vi "RGseriesSeria210216Ceramic.vi"() -> ()   [LabVIEW 2015]
uses:
  <vilib>/Instr/_visa.llb/VISA Configure Serial Port (Instr).vi
  <userlib>/caLab/Private/Get_PV-1D.vi
  <userlib>/caLab/Private/Get_PV.vi
  <userlib>/caLab/Private/Put_DBL-1D_PV-1D.vi
panel:
  out "read buffer 2":string
  out "read buffer":string
  out "concatenated string":string
  out "ReadWait":i16
  out "WriteWait":i16
  in  "Ifactor":dbl=33.3
  in  "APX:PS2_T_RV":dbl
  out "APX:PS2_V_EV":dbl format="%.3f"
  out "APX:PS2_I_EV":dbl format="%.3f"
  out "Ilim_factor":dbl
  out "Vlim_factor":dbl
  out "SSE:Tsample":dbl
  in  "I lower limit":dbl
  in  "V lower limit":dbl
  in  "I upper limit":dbl=2.8
  in  "V upper limit":dbl=18.0
  out "APX:PS2_Ct":dbl
  out "APX:PS2_Rzero":dbl
  in  "Heater":u16(ring) items=["Ceramic W/Mo", "Kanthal A-1"]
  out "APX:Theater":dbl
  out "APX:PS2_R_MV":dbl format="%.2f"
  out "PS1:R_MV":dbl format="%.2f"
  out "APX:Tpiezo":dbl
  in  "REMOTE/LOCAL":bool
  out "APX:Tcopper":dbl
  in  "Timer1":bool
  in  "Reset Timer1":bool=TRUE caption="Auto Reset"
  out "Time has Elapsed":bool
  in  "Time Target1 (min)":dbl=1.0 caption="Time Target (s)"
  out "Elapsed Time (min)":dbl caption="Elapsed Time (s)"
  in  "PS1:I_RV":dbl min=0.0 max=0.5 step=0.01
  in  "PS1:V_RV":dbl min=0.0 max=5.0 step=0.01
  out "PS1:P_MV":dbl format="%.2f"
  out "PS1:I_MV":dbl format="%.3g"
  out "PS1:V_MV":dbl format="%.3g"
  in  "PS1:OUT":bool
  out "APX:Thpc OK?":bool
  out "APX:Tpiezo OK?":bool
  out "PS2_P_MV":dbl format="%.2f"
  in  "APX:PS2_I_RV":dbl min=0.0 max=0.5 step=0.002
  in  "APX:PS2_OUT":bool
  in  "stop":bool
  out "APX:PS2_I_MV":dbl format="%.3g"
  out "APX:PS2_V_MV":dbl format="%.3g"
  in  "VISA resource name":refnum<visa-resource-name>="COM12"
  in  "APX:PS2_V_RV":dbl min=0.0 max=8.0 step=0.05
  # "COM20"
  # "#2"
  # "Sample Heater Control"
  # "Copper mesh temperature control"
  # "COM12"
  # "V"
  # "V"
  # "A"
  # "A"
  # "Max 1.2A/0.4x0.1wire"
  # "W"
  # "ohm"
  # "W"
  # "ohm"
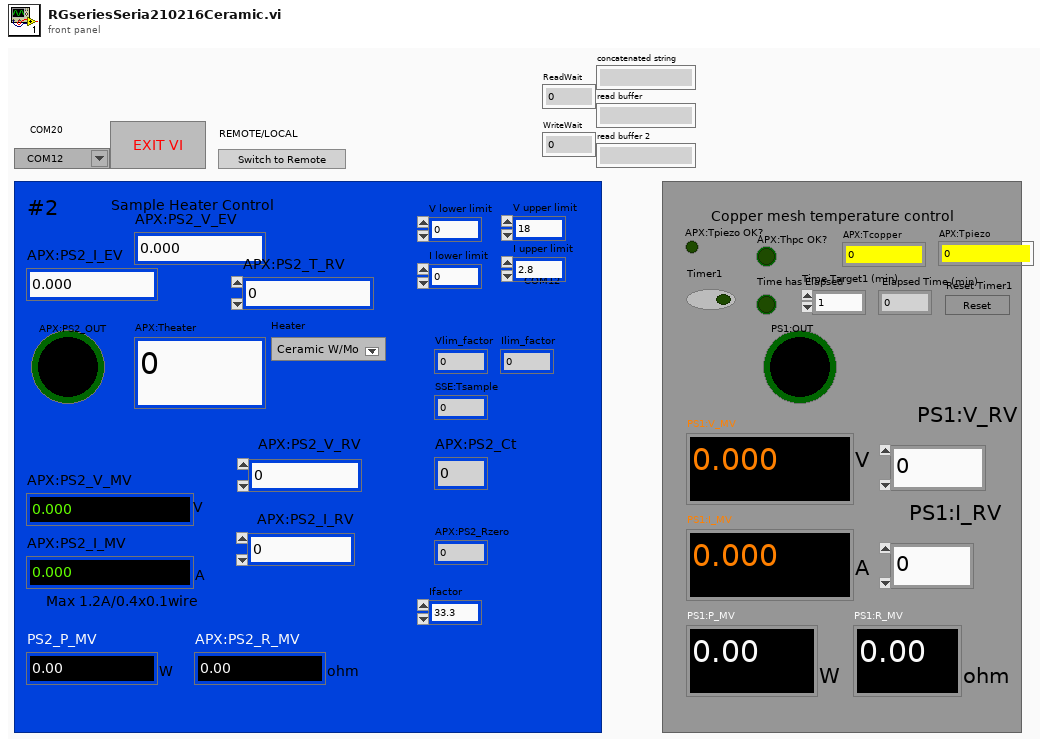
[diagram p1: front panel]
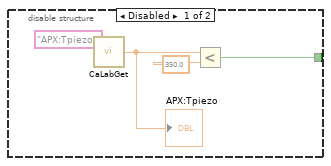
[diagram p2: hidden frame]
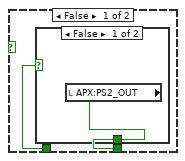
[diagram p4: hidden frame]
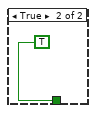
[diagram p5: hidden frame]
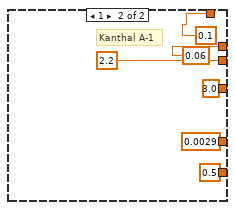
[diagram p6: hidden frame]
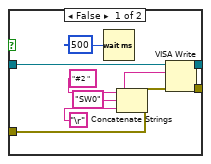
[diagram p7: hidden frame]
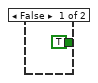
[diagram p9: hidden frame]
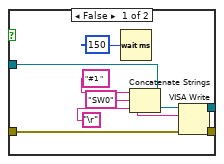
[diagram p10: hidden frame]
diagram:
  w54 = u16 0 items=["None", "XON/XOFF", "RTS/CTS", "XON/XOFF & RTS/CTS", "DTR/DSR", "XON/XOFF & DTR/DSR"] ("flow control (0:none)")
  w55 = u16 10 items=["1.0"=10, "1.5"=15, "2.0"=20] ("stop bits (10: 1 bit)")
  # "enable output"
  # "disable remote control"
  # "OpenComport"
  # "Stop bits"
  # "enable remote control"
  # "enable output"
  n1 = Concatenate Strings("#2 " ("initial string"), "REN" ("string"), "\r") -> (w53:string)
  n2 = call-poly "VISA Configure Serial Port"("VISA resource name"=refnum<visa-resource-name> "COM20", "timeout (10sec)"=u32 10000, "baud rate (9600)"=u32 9600, "data bits (8)"=u16 8, "parity (0:none)"=enum16{"None", "Odd", "Even", "Mark", "Space"}."None", "stop bits (10: 1 bit)"=w55, "flow control (0:none)"=w54) -> ("VISA resource name out"=w4:refnum<visa-resource-name>, "error out"=w3:errorcluster)  [unwired: 7 in]
  n3 = VISA Clear(VISA resource name=w4, error in (no error)=w3) -> (VISA resource name out=w1:refnum<visa-resource-name>, error out=w2:errorcluster)
  n4 = VISA Write(VISA resource name=w1, write buffer=w53, error in (no error)=w2) -> (VISA resource name out=w27:refnum<visa-resource-name>, error out=w20:errorcluster)  [unwired: 1 out]
  n5 = flat-sequence {
    tunnel: w20 -> [w68]
    tunnel: [w68] -> w21
    frame #0 {
      n6 = Wait (ms)(milliseconds to wait=u32 500) -> ()  [unwired: 1 out]
    }
  }
  n7 = Concatenate Strings("#1 " ("initial string"), "REN" ("string"), "\r") -> (w22:string)
  n8 = flat-sequence {
    frame #0 {
      "WriteWait" <- i16 200 ("WriteWait")
      "ReadWait" <- i16 200 ("ReadWait")
    }
  }
  n9 = VISA Write(VISA resource name=w27, write buffer=w22, error in (no error)=w21) -> (VISA resource name out=w26:refnum<visa-resource-name>, error out=w19:errorcluster)  [unwired: 1 out]
  n10 = flat-sequence {
    tunnel: [w74] -> w40
    tunnel: w19 -> [w74]
    frame #0 {
      n11 = Wait (ms)(milliseconds to wait=u32 500) -> ()  [unwired: 1 out]
      n12 = property on="APX:PS2_V_RV" class="DigNum (strict)"("Value"=0.0 ("VCN_REQ")) -> ()  [unwired: 2 in, 2 out]
      n13 = property on="APX:PS2_I_RV" class="DigNum (strict)"("Value"=0.0 ("APX:RG183_I_RV")) -> ()  [unwired: 2 in, 2 out]
    }
  }
  n14 = local write "REMOTE/LOCAL"(FALSE ("REMOTE/LOCAL")) -> ()
  n15 = Concatenate Strings("#2 " ("format string"), "SW0" ("initial string"), "\r" ("input 1")) -> (w52:string)
  n16 = VISA Write(VISA resource name=w26, write buffer=w52, error in (no error)=w40) -> (VISA resource name out=w42:refnum<visa-resource-name>, error out=w41:errorcluster)  [unwired: 1 out]
  n17 = while {
    tunnel: w42 -> [w84]
    tunnel: w41 -> [w85]
    tunnel: [w81] -> w39
    tunnel: [w80] -> w38
    stop <- "stop" stop-if-true
    n18 = flat-sequence {
      tunnel: w84 -> [w89]
      tunnel: w85 -> [w87]
      tunnel: [w86] -> w78
      tunnel: [w88] -> w77
      tunnel: [w198] -> w83
      tunnel: [w197] -> w82
      tunnel: w78 -> [w156]
      tunnel: w77 -> [w157]
      tunnel: w83 -> [w366]
      tunnel: w82 -> [w363]
      tunnel: [w348] -> w76
      tunnel: [w347] -> w75
      tunnel: [w442] -> w80
      tunnel: [w443] -> w81
      tunnel: w76 -> [w443]
      tunnel: w75 -> [w442]
      frame #0 {
        n19 = disable-structure shown="Enabled" {
          disable-tunnel: [w99 TRUE ("APX:Tpiezo OK?")] -> w92
          frame Disabled {
            n20 = call-poly "CaLabGet.vi"("PV Name"="APX:Tpiezo") -> ("1rst Value (number)"=w101:dbl)  [unwired: 8 in, 6 out]
            "APX:Tpiezo" <- w101
            n21 = Less?(x=w101, y=350.0) -> (x < y?=w99:bool)
          }
          frame Enabled {
          }
        }
        "APX:Tpiezo OK?" <- w92
        n22 = case shown="0, Default" "Heater" {
          tunnel: [0.00483 ("APX:PS2_Ct") 0.0029 ("APX:PS2_Ct")] -> w95
          tunnel: [9.3 ("APX:PS2_Rzero") 0.5 ("APX:PS2_Rzero")] -> w96
          tunnel: [0.5 2.2] -> w97
          tunnel: [10.0 3.0] -> w98
          tunnel: [0.1 0.1] -> w91
          tunnel: [0.06 0.06] -> w90
          frame 0, Default {
            (unwired) 9.89 ("APX:PS2_Rzero")
            (unwired) 0.0325 ("APX:PS2_Ct")
            (unwired) 6.21 ("APX:PS2_Rzero")
            # "W/Mo"
          }
          frame 1 {
            # "Kanthal A-1"
          }
        }
        n23 = VISA Clear(VISA resource name=w89, error in (no error)=w87) -> (VISA resource name out=w88:refnum<visa-resource-name>, error out=w86:errorcluster)
        n24 = case shown="True" "REMOTE/LOCAL" {
          frame False {
          }
          frame True {
            w106 = 0 ("disabled index (col)")
            (unwired) "APX:Thpc"
            n25 = call-poly "CaLabGet.vi"("PV Names"=string[] ["APX:PS2_V_RV", "APX:PS2_I_RV", "APX:PS2_OUT_1", "APX:PS2_OUT_0", "SSE:Tsample"]) -> ("Value Array (number)"=w105:dbl[][])  [unwired: 8 in, 6 out]
            n26 = Index Array(array=w105, index (row)=4, index (col)=w106) -> (element=→"SSE:Tsample":dbl)
            n27 = Index Array(array=w105, index (row)=2, index (col)=w106) -> (element=w119:dbl)
            n28 = Index Array(array=w105, index (row)=0, index (col)=w106) -> (element=w109:dbl)
            n29 = Index Array(array=w105, index (row)=1, index (col)=w106) -> (element=w108:dbl)
            n30 = Index Array(array=w105, index (row)=3 ("disabled index (row)"), index (col)=w106) -> (element=w113:dbl)
            n31 = Number To Boolean Array(number=w119) -> (Boolean array=w118:bool[])
            n32 = Number To Boolean Array(number=w113) -> (Boolean array=w115:bool[])
            n33 = local write "APX:PS2_I_RV"(w108) -> ()
            n34 = Index Array(array=w118, index=0) -> (element=w111:bool)
            n35 = local write "APX:PS2_V_RV"(w109) -> ()
            n36 = Index Array(array=w115, index=0) -> (element=w112:bool)
            n37 = case shown="True" w112 {
              tunnel: w111 -> [w125 _]
              tunnel: [w124 FALSE] -> w110
              frame False {
                n38 = case shown="False" w125 {
                  tunnel: [w126 TRUE] -> w124
                  frame False {
                    n39 = local read "APX:PS2_OUT"() -> (w126:bool)
                  }
                  frame True {
                  }
                }
              }
              frame True {
              }
            }
            n40 = local write "APX:PS2_OUT"(w110) -> ()
          }
        }
        n41 = local write "I upper limit"(w97) -> ()
        n42 = local write "V upper limit"(w98) -> ()
        n43 = local write "APX:PS2_Ct"(w95) -> ()
        n44 = local write "APX:PS2_Rzero"(w96) -> ()
        n45 = local write "V lower limit"(w91) -> ()
        n46 = local write "I lower limit"(w90) -> ()
      }
      frame #1 {
        w172 = 293.0 ("y")
        # "measure current"
        # "measure voltage"
        # "measure voltage"
        # "measure curent"
        # "Measured Voltage"
        # "Measured Current"
        # "Set current"
        # "Set voltage"
        # "disable output"
        n47 = local read "APX:PS2_Rzero"() -> (w167:dbl)
        n48 = local read "APX:PS2_R_MV"() -> (w185:dbl)
        n49 = In Range and Coerce(upper limit=65.0, x=w185, lower limit=w167) -> (coerced(x)=w183:dbl)  [unwired: 1 out]
        n50 = Divide(x=w183, y=w167) -> (x/y=w182:dbl)
        n51 = Subtract(x="APX:PS2_T_RV", y=w172) -> (x-y=w166:dbl)
        n52 = Subtract(x=w182, y=1.0) -> (x-y=w180:dbl)
        n53 = local read "APX:PS2_Ct"() -> (w171:dbl)
        n54 = Multiply(x=w166, y=w171) -> (x*y=w170:dbl)
        n55 = Divide(x=w180, y=w171) -> (x/y=w179:dbl)
        n56 = Add(x=w170, y=1.0) -> (x+y=w168:dbl)
        n57 = Multiply(x=w168, y=w167) -> (x*y=w163:dbl)
        n58 = Multiply(x=w166, y=0.02) -> (x*y=w162:dbl)
        "APX:PS2_V_EV" <- w162
        n59 = flat-sequence {
          tunnel: w157 -> [w259]
          tunnel: w156 -> [w258]
          tunnel: [w259] -> w154
          tunnel: [w258] -> w155
          tunnel: [w257] -> w151
          frame #0 {
            n60 = local read "WriteWait"() -> (w257:i16)
            n61 = Wait (ms)(milliseconds to wait=w257) -> ()  [unwired: 1 out]
          }
        }
        n62 = Add(x=w179, y=w172) -> (x+y=→"APX:Theater":dbl)
        n63 = Divide(x=w162, y=w163) -> (x/y=→"APX:PS2_I_EV":dbl)
        n64 = case shown="True" "APX:PS2_OUT" {
          tunnel: w154 -> [w269 w278]
          tunnel: w155 -> [w268 w277]
          tunnel: [w267 w276] -> w196
          tunnel: [w266 w275] -> w195
          frame False {
            n65 = Wait (ms)(milliseconds to wait=u32 500) -> ()  [unwired: 1 out]
            n66 = Concatenate Strings("#2 " ("format string"), "SW0" ("initial string"), "\r" ("input 1")) -> (w271:string)
            n67 = VISA Write(VISA resource name=w269, write buffer=w271, error in (no error)=w268) -> (VISA resource name out=w266:refnum<visa-resource-name>, error out=w267:errorcluster)  [unwired: 1 out]
          }
          frame True {
            n68 = Concatenate Strings("#2 " ("format string"), "SW1" ("initial string"), "\r" ("input 1")) -> (w279:string)
            n69 = VISA Write(VISA resource name=w278, write buffer=w279, error in (no error)=w277) -> (VISA resource name out=w275:refnum<visa-resource-name>, error out=w276:errorcluster)  [unwired: 1 out]
          }
        }
        n70 = flat-sequence {
          tunnel: w195 -> [w296]
          tunnel: w196 -> [w297]
          tunnel: [w297] -> w199
          tunnel: [w296] -> w200
          tunnel: w151 -> [w295]
          frame #0 {
            n71 = Wait (ms)(milliseconds to wait=w295) -> ()  [unwired: 1 out]
          }
        }
        n72 = In Range and Coerce(upper limit="V upper limit", x="APX:PS2_V_RV", lower limit="V lower limit") -> (coerced(x)=w193:dbl)  [unwired: 1 out]
        n73 = Multiply(x=5.5, y=w193) -> (x*y=w254:dbl)
        n74 = Number To Fractional String(number=w254, width (-)=i16 5, precision (6)=i16 2) -> (F-format string=w255:string)  [unwired: 1 in]
        n75 = Concatenate Strings("#2" ("format string"), "VCN " ("initial string"), w255, "\r") -> (w204:string)
        "concatenated string" <- w204
        n76 = VISA Write(VISA resource name=w200, write buffer=w204, error in (no error)=w199) -> (VISA resource name out=w161:refnum<visa-resource-name>, error out=w160:errorcluster)  [unwired: 1 out]
        n77 = local read "ReadWait"() -> (w141:i16)
        n78 = Concatenate Strings("#2 " ("format string"), "VM" ("initial string"), "\r" ("input 1")) -> (w231:string)
        n79 = flat-sequence {
          tunnel: w161 -> [w265]
          tunnel: w160 -> [w264]
          tunnel: [w265] -> w150
          tunnel: [w264] -> w148
          tunnel: [w263] -> w153
          tunnel: w141 -> [w263]
          frame #0 {
            n80 = Wait (ms)(milliseconds to wait=w263) -> ()  [unwired: 1 out]
          }
        }
        n81 = VISA Clear(VISA resource name=w150, error in (no error)=w148) -> (VISA resource name out=w149:refnum<visa-resource-name>, error out=w147:errorcluster)
        n82 = VISA Write(VISA resource name=w149, write buffer=w231, error in (no error)=w147) -> (VISA resource name out=w220:refnum<visa-resource-name>, error out=w218:errorcluster)  [unwired: 1 out]
        n83 = flat-sequence {
          tunnel: w220 -> [w294]
          tunnel: [w294] -> w219
          tunnel: w218 -> [w293]
          tunnel: [w293] -> w217
          tunnel: [w292] -> w142
          tunnel: w141 -> [w292]
          frame #0 {
            n84 = Wait (ms)(milliseconds to wait=w292) -> ()  [unwired: 1 out]
          }
        }
        n85 = In Range and Coerce(upper limit="I upper limit", x="APX:PS2_I_RV", lower limit="I lower limit") -> (coerced(x)=w191:dbl)  [unwired: 1 out]
        n86 = Multiply(x=33.0, y=w191) -> (x*y=w244:dbl)
        n87 = property class="Instr"(reference=w219, error in=w217) -> (reference out=w226:refnum<visa-resource-name>, error out=w225:errorcluster, "Serial Settings:Number of Bytes at Serial Port"=w224:u32)
        n88 = Number To Fractional String(number=w244, width (-)=i16 5, precision (6)=i16 2) -> (F-format string=w247:string)  [unwired: 1 in]
        n89 = VISA Read(VISA resource name=w226, byte count=w224, error in (no error)=w225) -> (VISA resource name out=w212:refnum<visa-resource-name>, read buffer=w205:string, error out=w211:errorcluster)  [unwired: 1 out]
        "read buffer" <- w205
        n90 = flat-sequence {
          tunnel: w212 -> [w288]
          tunnel: w211 -> [w287]
          tunnel: [w288] -> w209
          tunnel: [w287] -> w210
          tunnel: w153 -> [w286]
          tunnel: [w286] -> w152
          frame #0 {
            n91 = Wait (ms)(milliseconds to wait=w286) -> ()  [unwired: 1 out]
          }
        }
        n92 = Concatenate Strings("#2 " ("initial string"), "ICN " ("initial string"), w247, "\r") -> (w203:string)
        n93 = String Subset(string=w205, offset (0)=3) -> (substring=w202:string)  [unwired: 1 in]
        n94 = Concatenate Strings("#2 " ("format string"), "IM" ("initial string"), "\r" ("input 1")) -> (w228:string)
        n95 = VISA Write(VISA resource name=w209, write buffer=w203, error in (no error)=w210) -> (VISA resource name out=w159:refnum<visa-resource-name>, error out=w158:errorcluster)  [unwired: 1 out]
        n96 = Fract/Exp String To Number(string=w202) -> (number=w240:dbl)  [unwired: 3 in, 1 out]
        n97 = flat-sequence {
          tunnel: w159 -> [w262]
          tunnel: [w262] -> w145
          tunnel: [w261] -> w146
          tunnel: w158 -> [w261]
          tunnel: w142 -> [w260]
          frame #0 {
            n98 = Wait (ms)(milliseconds to wait=w260) -> ()  [unwired: 1 out]
          }
        }
        n99 = Divide(x=w240, y=5.5 ("x")) -> (x/y=w188:dbl)
        "APX:PS2_V_MV" <- w188
        n100 = flat-sequence {
          tunnel: w216 -> [w291]
          tunnel: w215 -> [w290]
          tunnel: [w291] -> w214
          tunnel: [w290] -> w213
          tunnel: w142 -> [w289]
          frame #0 {
            n101 = Wait (ms)(milliseconds to wait=w289) -> ()  [unwired: 1 out]
          }
        }
        n102 = VISA Clear(VISA resource name=w145, error in (no error)=w146) -> (VISA resource name out=w143:refnum<visa-resource-name>, error out=w144:errorcluster)
        n103 = VISA Write(VISA resource name=w143, write buffer=w228, error in (no error)=w144) -> (VISA resource name out=w216:refnum<visa-resource-name>, error out=w215:errorcluster)  [unwired: 1 out]
        n104 = property class="Instr"(reference=w214, error in=w213) -> (reference out=w223:refnum<visa-resource-name>, error out=w222:errorcluster, "Serial Settings:Number of Bytes at Serial Port"=w221:u32)
        n105 = VISA Read(VISA resource name=w223, byte count=w221, error in (no error)=w222) -> (VISA resource name out=w208:refnum<visa-resource-name>, read buffer=w206:string, error out=w207:errorcluster)  [unwired: 1 out]
        "read buffer 2" <- w206
        n106 = flat-sequence {
          tunnel: w208 -> [w285]
          tunnel: w207 -> [w284]
          tunnel: [w285] -> w198
          tunnel: [w284] -> w197
          tunnel: w152 -> [w283]
          frame #0 {
            n107 = Wait (ms)(milliseconds to wait=w283) -> ()  [unwired: 1 out]
          }
        }
        n108 = String Subset(string=w206, offset (0)=3) -> (substring=w201:string)  [unwired: 1 in]
        n109 = Fract/Exp String To Number(string=w201) -> (number=w237:dbl)  [unwired: 3 in, 1 out]
        n110 = Divide(x=w237, y=33.5 ("x")) -> (x/y=w189:dbl)
        "APX:PS2_I_MV" <- w189
        n111 = Multiply(x=w188, y=w189) -> (x*y=→"PS2_P_MV":dbl)
        n112 = Divide(x=w188, y=w189) -> (x/y=→"APX:PS2_R_MV":dbl)
      }
      frame #2 {
        (unwired) 33.3 ("x")
        (unwired) 37.35 ("x")
        # "measure voltage"
        # "Set voltage"
        # "measure curent"
        # "Measured Voltage"
        # "Measured Current"
        # "disable output"
        # "measure current"
        # "measure voltage"
        # "Set current"
        n113 = case shown="True" "Reset Timer1" {
          frame False {
          }
          frame True {
            n114 = property on="Elapsed Time (min)" class="DigNum (strict)"("Value"=0.0 ("Elapsed Time (min)")) -> ()  [unwired: 2 in, 2 out]
          }
        }
        n115 = case shown="True" "Timer1" {
          tunnel: "Time Target1 (min)" -> [_ w400]
          tunnel: [TRUE w399] -> w302
          frame False {
          }
          frame True {
            w404 = 60.0 ("y")
            n116 = Multiply(x=w400, y=w404) -> (x*y=w402:dbl)
            n117 = call "Elapsed Time"("Time Target (s)"=w402) -> ("Elapsed Time (s)"=w403:dbl, "Time has Elapsed"=w401:bool)  [unwired: 11 in, 6 out]
            "Time has Elapsed" <- w401
            n118 = Divide(x=w403, y=w404) -> (x/y=→"Elapsed Time (min)":dbl)
            n119 = Not(x=w401) -> (.not. x?=w399:bool)
          }
        }
        n120 = call-poly "CaLabGet.vi"("PV Name"="APX:Tcopper") -> ("1rst Value (number)"=w392:dbl)  [unwired: 8 in, 6 out]
        "APX:Tcopper" <- w392
        n121 = Less?(x=w392, y=420.0) -> (x < y?=w365:bool)
        "APX:Thpc OK?" <- w365
        n122 = disable-structure shown="Disabled" {
          frame Disabled {
            n123 = Wait (ms)(milliseconds to wait=u32 200) -> ()  [unwired: 1 out]
          }
          frame Enabled {
          }
        }
        n124 = And(x=w365, y="PS1:OUT") -> (x .and. y?=w342:bool)
        n125 = And(x=w342, y=w302) -> (x .and. y?=w305:bool)
        n126 = case shown="True" w305 {
          tunnel: w366 -> [w409 w418]
          tunnel: w363 -> [w408 w417]
          tunnel: [w407 w416] -> w309
          tunnel: [w406 w415] -> w308
          frame False {
            n127 = Wait (ms)(milliseconds to wait=u32 150) -> ()  [unwired: 1 out]
            n128 = Concatenate Strings("#1 " ("format string"), "SW0" ("initial string"), "\r" ("input 1")) -> (w413:string)
            n129 = VISA Write(VISA resource name=w409, write buffer=w413, error in (no error)=w408) -> (VISA resource name out=w406:refnum<visa-resource-name>, error out=w407:errorcluster)  [unwired: 1 out]
          }
          frame True {
            n130 = Concatenate Strings("#1 " ("format string"), "SW1" ("initial string"), "\r" ("input 1")) -> (w422:string)
            n131 = VISA Write(VISA resource name=w418, write buffer=w422, error in (no error)=w417) -> (VISA resource name out=w415:refnum<visa-resource-name>, error out=w416:errorcluster)  [unwired: 1 out]
          }
        }
        n132 = local read "WriteWait"() -> (w331:i16)
        n133 = In Range and Coerce(upper limit=5.01, x="PS1:V_RV", lower limit=0.0) -> (coerced(x)=w321:dbl)  [unwired: 1 out]
        n134 = flat-sequence {
          tunnel: [w425] -> w306
          tunnel: w309 -> [w425]
          tunnel: [w424] -> w307
          tunnel: w308 -> [w424]
          tunnel: w331 -> [w423]
          frame #0 {
            n135 = Wait (ms)(milliseconds to wait=w423) -> ()  [unwired: 1 out]
          }
        }
        n136 = Multiply(x=5.55, y=w321) -> (x*y=w312:dbl)
        n137 = Number To Fractional String(number=w312, width (-)=i16 5, precision (6)=i16 2) -> (F-format string=w311:string)  [unwired: 1 in]
        n138 = Concatenate Strings("#1" ("format string"), "VCN " ("initial string"), w311, "\r") -> (w326:string)
        n139 = Concatenate Strings("#1" ("format string"), "VM" ("initial string"), "\r" ("input 1")) -> (w325:string)
        n140 = VISA Write(VISA resource name=w307, write buffer=w326, error in (no error)=w306) -> (VISA resource name out=w301:refnum<visa-resource-name>, error out=w300:errorcluster)  [unwired: 1 out]
        n141 = flat-sequence {
          tunnel: w301 -> [w396]
          tunnel: [w397] -> w299
          tunnel: w300 -> [w397]
          tunnel: [w396] -> w298
          tunnel: w331 -> [w395]
          frame #0 {
            n142 = Wait (ms)(milliseconds to wait=w395) -> ()  [unwired: 1 out]
          }
        }
        n143 = VISA Write(VISA resource name=w298, write buffer=w325, error in (no error)=w299) -> (VISA resource name out=w327:refnum<visa-resource-name>, error out=w328:errorcluster)  [unwired: 1 out]
        n144 = local read "ReadWait"() -> (w332:i16)
        n145 = property class="Instr"(reference=w329, error in=w330) -> (reference out=w387:refnum<visa-resource-name>, error out=w388:errorcluster, "Serial Settings:Number of Bytes at Serial Port"=w389:u32)
        n146 = flat-sequence {
          tunnel: w327 -> [w428]
          tunnel: [w428] -> w329
          tunnel: w328 -> [w427]
          tunnel: [w427] -> w330
          tunnel: w332 -> [w426]
          frame #0 {
            n147 = Wait (ms)(milliseconds to wait=w426) -> ()  [unwired: 1 out]
          }
        }
        n148 = VISA Read(VISA resource name=w387, byte count=w389, error in (no error)=w388) -> (VISA resource name out=w346:refnum<visa-resource-name>, read buffer=w390:string, error out=w344:errorcluster)  [unwired: 1 out]
        n149 = flat-sequence {
          tunnel: w346 -> [w435]
          tunnel: [w435] -> w345
          tunnel: [w434] -> w343
          tunnel: w344 -> [w434]
          tunnel: w331 -> [w433]
          frame #0 {
            n150 = Wait (ms)(milliseconds to wait=w433) -> ()  [unwired: 1 out]
          }
        }
        n151 = String Subset(string=w390, offset (0)=3) -> (substring=w380:string)  [unwired: 1 in]
        n152 = In Range and Coerce(upper limit=0.501, x="PS1:I_RV", lower limit=0.0) -> (coerced(x)=w384:dbl)  [unwired: 1 out]
        n153 = Fract/Exp String To Number(string=w380) -> (number=w374:dbl)  [unwired: 3 in, 1 out]
        n154 = Multiply(x="Ifactor", y=w384) -> (x*y=w370:dbl)
        n155 = Number To Fractional String(number=w370, width (-)=i16 5, precision (6)=i16 2) -> (F-format string=w368:string)  [unwired: 1 in]
        n156 = Concatenate Strings("#1 " ("initial string"), "ICN " ("initial string"), w368, "\r") -> (w385:string)
        n157 = VISA Write(VISA resource name=w345, write buffer=w385, error in (no error)=w343) -> (VISA resource name out=w336:refnum<visa-resource-name>, error out=w334:errorcluster)  [unwired: 1 out]
        n158 = flat-sequence {
          tunnel: w336 -> [w431]
          tunnel: [w431] -> w335
          tunnel: w334 -> [w430]
          tunnel: [w430] -> w333
          tunnel: w331 -> [w429]
          frame #0 {
            n159 = Wait (ms)(milliseconds to wait=w429) -> ()  [unwired: 1 out]
          }
        }
        n160 = Concatenate Strings("#1 " ("format string"), "IM" ("initial string"), "\r" ("input 1")) -> (w386:string)
        n161 = VISA Write(VISA resource name=w335, write buffer=w386, error in (no error)=w333) -> (VISA resource name out=w351:refnum<visa-resource-name>, error out=w350:errorcluster)  [unwired: 1 out]
        n162 = flat-sequence {
          tunnel: w351 -> [w441]
          tunnel: w350 -> [w440]
          tunnel: [w441] -> w357
          tunnel: [w440] -> w356
          tunnel: w332 -> [w439]
          frame #0 {
            n163 = Wait (ms)(milliseconds to wait=w439) -> ()  [unwired: 1 out]
          }
        }
        n164 = property class="Instr"(reference=w357, error in=w356) -> (reference out=w360:refnum<visa-resource-name>, error out=w359:errorcluster, "Serial Settings:Number of Bytes at Serial Port"=w358:u32)
        n165 = VISA Read(VISA resource name=w360, byte count=w358, error in (no error)=w359) -> (VISA resource name out=w355:refnum<visa-resource-name>, read buffer=w353:string, error out=w354:errorcluster)  [unwired: 1 out]
        n166 = flat-sequence {
          tunnel: w355 -> [w438]
          tunnel: w354 -> [w437]
          tunnel: [w438] -> w348
          tunnel: [w437] -> w347
          tunnel: w331 -> [w436]
          frame #0 {
            n167 = Wait (ms)(milliseconds to wait=w436) -> ()  [unwired: 1 out]
          }
        }
        n168 = String Subset(string=w353, offset (0)=3) -> (substring=w352:string)  [unwired: 1 in]
        n169 = Fract/Exp String To Number(string=w352) -> (number=w362:dbl)  [unwired: 3 in, 1 out]
        n170 = Divide(x=w374, y=5.55 ("x")) -> (x/y=w340:dbl)
        "PS1:V_MV" <- w340
        n171 = Divide(x=w362, y="Ifactor") -> (x/y=w339:dbl)
        "PS1:I_MV" <- w339
        n172 = Divide(x=w340, y=w339) -> (x/y=→"PS1:R_MV":dbl)
        n173 = Multiply(x=w340, y=w339) -> (x*y=→"PS1:P_MV":dbl)
      }
      frame #3 {
        n174 = flat-sequence {
          frame #0 {
            w448 = 0.0 ("element")
            n175 = local read "APX:PS2_OUT"() -> (w452:bool)
            n176 = local read "APX:PS2_R_MV"() -> (w457:dbl)
            n177 = local read "APX:PS2_V_MV"() -> (w455:dbl)
            n178 = local read "APX:PS2_I_MV"() -> (w456:dbl)
            n179 = local read "APX:Theater"() -> (w458:dbl)
            n180 = Boolean To (0,1)(Boolean=w452) -> (0, 1=w451:i16)
            n181 = local read "APX:PS2_Rzero"() -> (w444:dbl)
            n182 = Build Array("APX:Theater", "APX:PS2_R_MV", "APX:PS2_I_MV", "APX:PS2_V_MV", "APX:PS2_OUT", "APX:PS2_OUT_0", "APX:PS2_OUT_1", "APX:PS2_Rzero", "APX:PS2_Ct") -> (w463:string[])
            n183 = local read "APX:PS2_Ct"() -> (w445:dbl)
            n184 = Build Array(w458, w457, w456, w455, w451, w448, w448, w444, w445) -> (w454:dbl[])
            n185 = call-poly <userlib>:"CaLabPut.vi"("Values"=w454, "PV Names"=w463) -> ()  [unwired: 6 in, 4 out]
          }
        }
      }
    }
  }
  n186 = Concatenate Strings("#2 " ("format string"), "SW0" ("initial string"), "\r" ("input 1")) -> (w46:string)
  n187 = VISA Write(VISA resource name=w39, write buffer=w46, error in (no error)=w38) -> (VISA resource name out=w16:refnum<visa-resource-name>, error out=w14:errorcluster)  [unwired: 1 out]
  n188 = flat-sequence {
    tunnel: w16 -> [w464]
    tunnel: w14 -> [w466]
    tunnel: [w464] -> w15
    tunnel: [w466] -> w13
    frame #0 {
      n189 = Wait (ms)(milliseconds to wait=u32 200) -> ()  [unwired: 1 out]
    }
  }
  n190 = Concatenate Strings("#2 " ("initial string"), "\r", "GTL" ("input 1")) -> (w51:string)
  n191 = VISA Write(VISA resource name=w15, write buffer=w51, error in (no error)=w13) -> (VISA resource name out=w8:refnum<visa-resource-name>, error out=w7:errorcluster)  [unwired: 1 out]
  n192 = flat-sequence {
    tunnel: w8 -> [w469]
    tunnel: w7 -> [w468]
    tunnel: [w469] -> w6
    tunnel: [w468] -> w5
    frame #0 {
      n193 = Wait (ms)(milliseconds to wait=u32 200) -> ()  [unwired: 1 out]
    }
  }
  n194 = Concatenate Strings("#1 " ("format string"), "SW0" ("initial string"), "\r" ("input 1")) -> (w33:string)
  n195 = VISA Write(VISA resource name=w6, write buffer=w33, error in (no error)=w5) -> (VISA resource name out=w12:refnum<visa-resource-name>, error out=w10:errorcluster)  [unwired: 1 out]
  n196 = flat-sequence {
    tunnel: w12 -> [w472]
    tunnel: w10 -> [w470]
    tunnel: [w472] -> w11
    tunnel: [w470] -> _
    tunnel: [w470] -> w9
    frame #0 {
      n197 = Wait (ms)(milliseconds to wait=u32 500) -> ()  [unwired: 1 out]
    }
  }
  n198 = Concatenate Strings("#1" ("initial string"), "\r", "GTL" ("input 1")) -> (w34:string)
  n199 = VISA Write(VISA resource name=w11, write buffer=w34, error in (no error)=w9) -> (VISA resource name out=w29:refnum<visa-resource-name>, error out=w28:errorcluster)  [unwired: 1 out]
  n200 = flat-sequence {
    tunnel: w29 -> [w477]
    tunnel: w28 -> [w476]
    tunnel: [w477] -> w48
    tunnel: [w476] -> w47
    frame #0 {
      n201 = Wait (ms)(milliseconds to wait=u32 500) -> ()  [unwired: 1 out]
      n202 = property on="APX:PS2_OUT" class="Bool (strict)"("Value"=FALSE ("Output")) -> ()  [unwired: 2 in, 2 out]
      n203 = property on="APX:PS2_V_RV" class="DigNum (strict)"("Value"=0.0 ("VCN_REQ")) -> ()  [unwired: 2 in, 2 out]
      n204 = property on="APX:PS2_I_RV" class="DigNum (strict)"("Value"=0.0 ("APX:RG183_I_RV")) -> ()  [unwired: 2 in, 2 out]
    }
  }
  n205 = VISA Close(VISA resource name=w48, error in (no error)=w47) -> ()  [unwired: 1 out]
